vi "OTP - Read Keys File.vi"(11 "File Path":path) -> (3 "keys":string[](array[string]))   [LabVIEW 2013]
panel:
  out "spreadsheet string":string
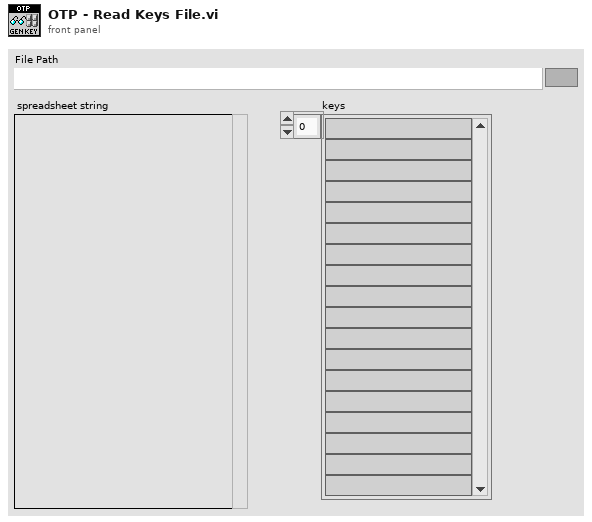
[diagram p1: front panel]
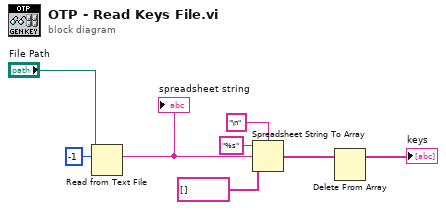
[diagram p0: block diagram]
diagram:
  n1 = Read from Text File(file (use dialog)="File Path", count=-1) -> (text=w6:string)  [unwired: 2 in, 3 out]
  "spreadsheet string" <- w6
  n2 = Spreadsheet String To Array(delimiter (Tab)="\n", format string="%s", spreadsheet string=w6, array type (2D Dbl)=string[] []) -> (array=w2:string[])
  n3 = Delete From Array(array=w2) -> (array with subset deleted=→"keys":string[])  [unwired: 2 in, 1 out]
